vi "Build and Transpose array.vi"() -> ()   [LabVIEW 2024]
panel:
  out "transposed array":dbl[][](array[numeric])
  out "2D array":dbl[][](array[numeric])
  in  "Array 2":dbl[][](array[numeric])
  in  "Array":dbl[](array[numeric])
  # "Overview:\nIn this Vi, we saw the usage of Build Array where the  \"Build Array\" function receives four constant inputs (1, 2, 3, and 4) and creates an array from them. \nThe array is then wired to an array indicator on the Front Panel. \nFunction palette->Array->Build Array"
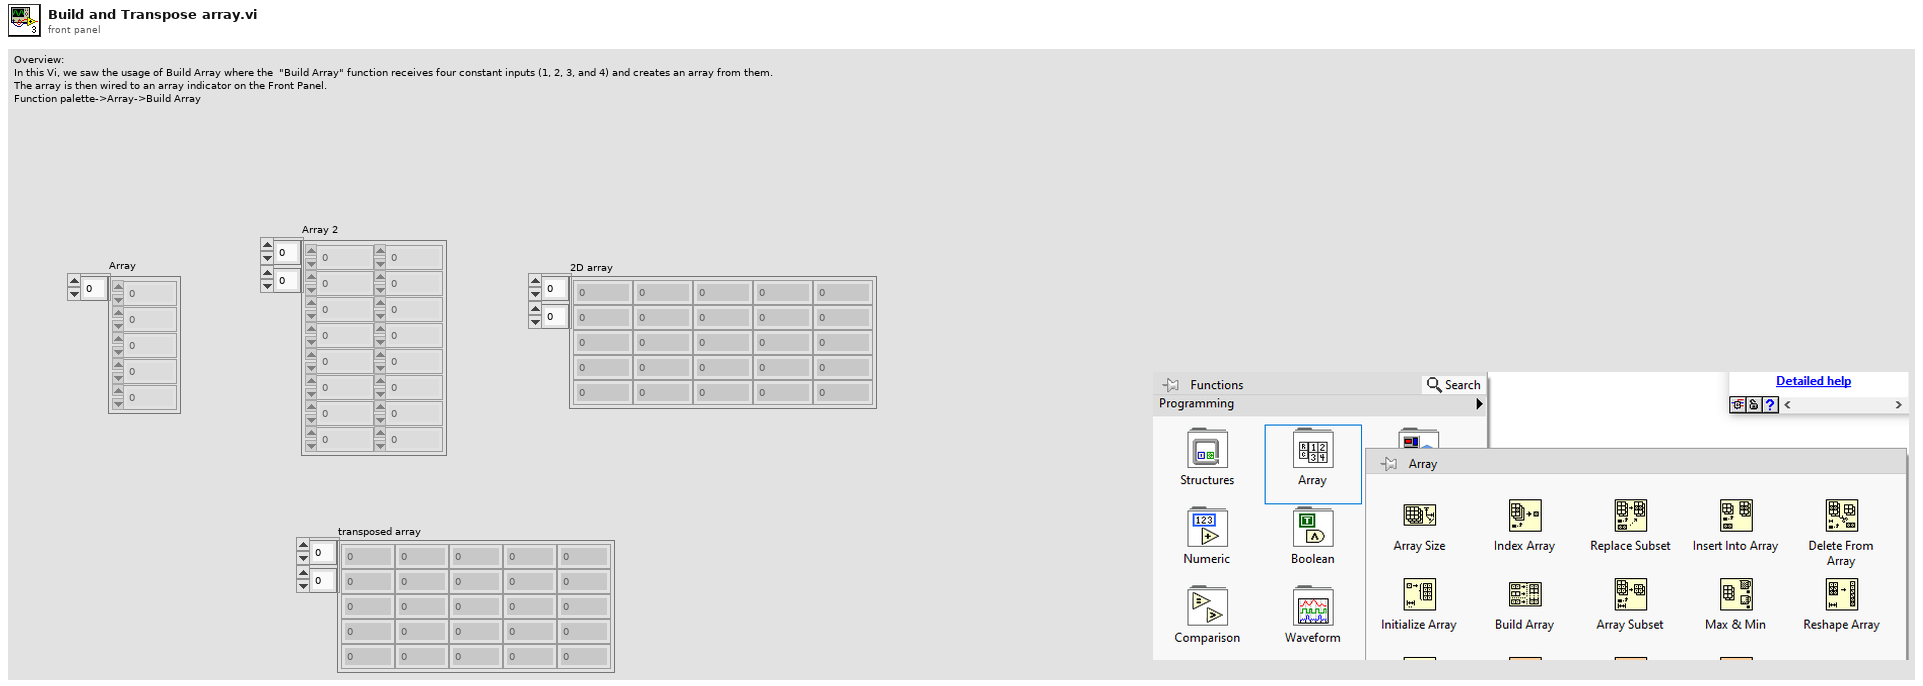
[diagram p1: front panel]
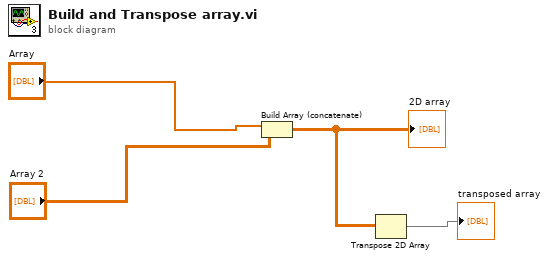
[diagram p0: block diagram]
diagram:
  n1 = Build Array (concatenate) "Build Array"("Array", "Array 2") -> (w2:dbl[][])
  "2D array" <- w2
  n2 = Transpose 2D Array(2D array=w2) -> (transposed array=→"transposed array":dbl[][])
